vi "Read Accelerometer.vi"(8 "Error In":errorcluster, 11 "EZ430-Chronos Ref":T2) -> (0 "Error Out":errorcluster, 2 "Accelerations":T1, 3 "EZ430-Chronos Config":T2)   [LabVIEW 2011, in "LVH-EZ430.lvlib"]
doc: "Read accelerometer data from the EZ430-Chronos. The watch must be transmitting in ACC mode before calling this VI."
uses:
  LVH-EZ430.lvlib
  Private/Type Defs/EZ430-Chronos Ref.ctl
  Private/Type Defs/Accelerations.ctl
  Private/Type Defs/Command.ctl
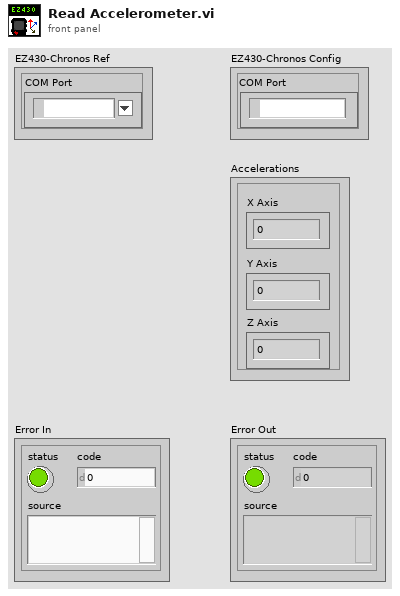
[diagram p1: front panel]
types:
  T1 = typedef "LVH-EZ430.lvlib/Accelerations.ctl" = cluster{"X Axis":i8, "Y Axis":i8, "Z Axis":i8}
  T2 = typedef "LVH-EZ430.lvlib/EZ430-Chronos Ref.ctl" = cluster{"COM Port":refnum<visa-resource-name>}
  T3 = typedef "LVH-EZ430.lvlib/Command.ctl" = enum8{"Get Hardware Status", "Reset RF Access Point", "Start BlueRobin Transmitter", "Set BlueRobin Trans ID", "Get BlueRobin Trans ID", "Set BlueRobin Heart Rate To Transmit", "Stop BlueRobin Transmitter", "Start ACC / PPT Mode", "Read ACC / PPT", "Stop SimpliciTI Stack"}
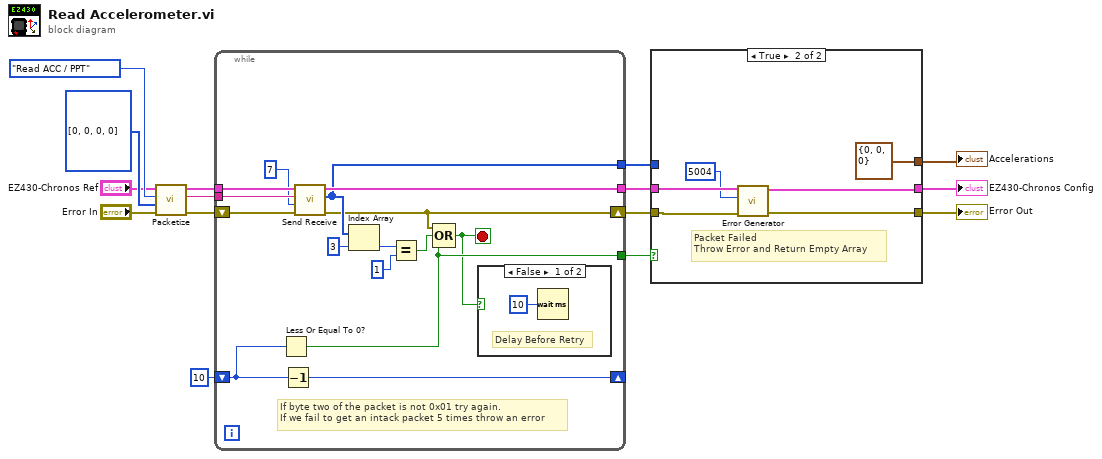
[diagram p0: block diagram]
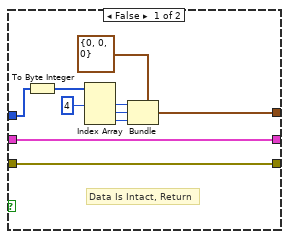
[diagram p2: hidden frame]
diagram:
  n1 = call "Packetize.vi"("Error In"="Error In", "Data"=u8[] [0, 0, 0, 0], "Command"=Command."Read ACC / PPT", "EZ430-Chronos Config"="EZ430-Chronos Ref") -> ("Error Out"=w11:errorcluster, "Packet"=w9:string, "EZ430-Chronos Config"=w10:T2)  [unwired: 5 in]
  n2 = while {
    tunnel: w10 -> [w29]
    tunnel: w9 -> [w28]
    tunnel: [w26] -> w4
    tunnel: [w23] -> w6
    shift-right: [w19] -> w2
    shift-left: w11 -> [w30]
    shift-right: [w24] -> _
    shift-left: 10 -> [w25]
    tunnel: [w17] -> w7
    stop <- w16 stop-if-true
    # "If byte two of the packet is not 0x01 try again.\nIf we fail to get an intack packet 5 times throw an error"
    n3 = Less Or Equal To 0?(x=w25) -> (x <= 0?=w17:bool)
    n4 = Decrement(x=w25) -> (x-1=w24:i32)
    n5 = call "Send Receive.vi"("Error In"=w30, "Bytes To Read"=u32 7, "Packet"=w28, "EZ430-Chronos Config"=w29) -> ("Error Out"=w19:errorcluster, "Data"=w23:u8[], "EZ430-Chronos Config"=w26:T2)  [unwired: 5 in]
    n6 = Index Array(array=w23, index=3) -> (element=w21:u8)
    n7 = Equal?(x=w21, y=u8 1) -> (x = y?=w18:bool)
    n8 = Compound Arithmetic op=OR(w19, w18, w17) -> (w16:bool)
    n9 = case shown="False" w16 {
      frame False {
        # "Delay Before Retry"
        n10 = Wait (ms)(milliseconds to wait=u32 10) -> ()  [unwired: 1 out]
      }
      frame True {
        # "Good Packet No \nNeed To Wait"
      }
    }
  }
  n11 = case shown="True" w7 {
    tunnel: w6 -> [w34 _]
    tunnel: [w41 w46] -> w5
    tunnel: w4 -> [w41 w47]
    tunnel: [w40 w45] -> w3
    tunnel: w2 -> [w40 w44]
    tunnel: [w33 T1 {"X Axis"=0, "Y Axis"=0, "Z Axis"=0} ("Accelerations")] -> w1
    frame False {
      # "Data Is Intact, Return"
      n12 = To Byte Integer(number=w34) -> (8bit integer=w35:i8[])
      n13 = Index Array(array=w35, index #1=4 ("index")) -> (element #1=w38:i8, element #2=w37:i8, element #3=w36:i8)  [unwired: 2 in]
      n14 = Bundle(cluster=T1 {"X Axis"=0, "Y Axis"=0, "Z Axis"=0} ("Accelerations"), "X Axis"=w38, "Y Axis"=w37, "Z Axis"=w36) -> (w33:T1)
    }
    frame True {
      # "Packet Failed\nThrow Error and Return Empty Array"
      n15 = call "Error Generator.vi"("Error In"=w44, "EZ430-Chronos Error Code"=5004, "EZ430-Chronos Ref"=w47) -> ("Error Out"=w45:errorcluster, "EZ430-Chronos Ref"=w46:T2)  [unwired: 7 in]
    }
  }
  "EZ430-Chronos Config" <- w5
  "Error Out" <- w3
  "Accelerations" <- w1
